vi "Get Response Fit.vi"(8 "error in (no error)":errorcluster, 11 "Head Impulse Fit in":refnum<class "Head Impulse Fit.lvclass">) -> (0 "error out":errorcluster, 2 "Fit out":dbl[](array[numeric]), 3 "Head Impulse Fit out":refnum<class "Head Impulse Fit.lvclass">)   [LabVIEW 2016, in "Head Impulse Fit.lvclass"]
uses:
  Head Impulse Fit.lvclass
  Head Impulse Fit.lvclass/Head Impulse Fit.ctl
  <vilib>/Analysis/1siggen.llb/Ramp Pattern by Samples.vi
  <vilib>/Analysis/polynomials.llb/1D Polynomial Evaluation (DBL).vi
  <vilib>/Analysis/NI_AALBase.lvlib
  <vilib>/Analysis/NI_AALPro.lvlib
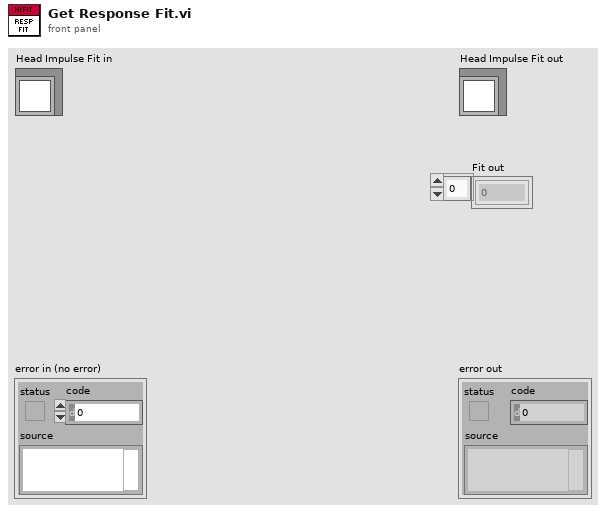
[diagram p1: front panel]
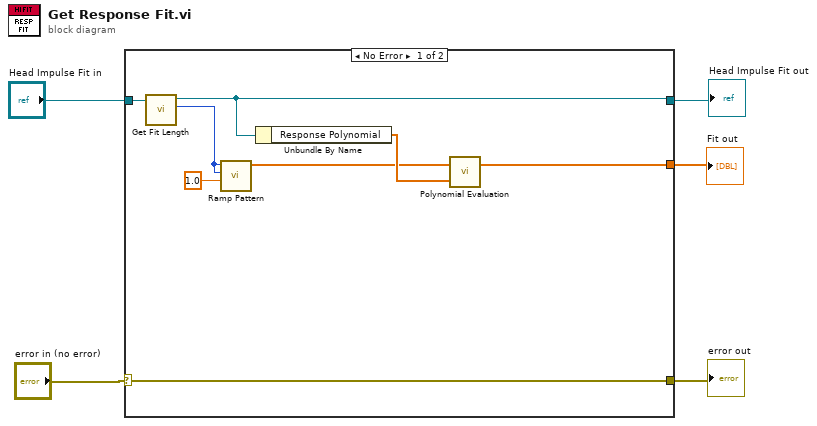
[diagram p0: block diagram]
diagram:
  n1 = case shown="No Error" "error in (no error)" {
    selector: "error in (no error)" -> [w13 w15]
    tunnel: "Head Impulse Fit in" -> [w12 w14]
    tunnel: [w9 w14] -> w1
    tunnel: [w13 w15] -> w3
    tunnel: [w6 _] -> w2
    frame No Error {
      n2 = call-dynamic "Get Fit Length.vi"("Abstract Fit in"=w12) -> ("Length"=w10:i32, "Abstract Fit out"=w9:refnum<class "Head Impulse Fit.lvclass">)  [unwired: 8 in, 1 out]
      n3 = call-poly <vilib>:"Ramp Pattern.vi"("start"=1.0, "end"=w10, "samples"=w10) -> ("Ramp Pattern"=w7:dbl[])  [unwired: 7 in, 1 out]
      n4 = Unbundle By Name(w9) -> ("Response Polynomial"=w8:dbl[])
      n5 = call-poly <vilib>:"Polynomial Evaluation.vi"("P(x)"=w8, "A"=w7) -> ("P(A)"=w6:dbl[])  [unwired: 1 out]
    }
    frame Error {
    }
  }
  "error out" <- w3
  "Head Impulse Fit out" <- w1
  "Fit out" <- w2
